vi "PCO_RecorderCopyImageCompressed.vi"(0 "phRec":u64, 1 "phCam":u64, 2 "dwImgIdx":u32, 3 "wRoiX0":u16, 4 "wRoiY0":u16, 5 "wRoiX1":u16, 6 "wRoiY1":u16, 7 "error in (no error)":errorcluster {"code" format="%x"}) -> (16 "strTimestamp":T2 {"lvTimestamp" format="%<%.6X\n%x>T"}, 17 "strMetadata":T1, 20 "phRec out":u64, 21 "ErrorMessage":i32 format="%x", 22 "bImgBuf":u8[][](array[numeric]), 23 "dwImgNumber":u32, 27 "error out":errorcluster {"code" format="%x"})   [LabVIEW 2020, in "Recorder.lvlib"]
doc: "int WINAPI PCO_RecorderCopyImageCompressed(HANDLE phRec, HANDLE phCam, DWORD dwImgIdx, WORD wRoiX0, WORD wRoiY0, WORD wRoiX1, WORD wRoiY1, BYTE* bImgBuf, DWORD* dwImgNumber,\n PCO_METADATA_STRUCT* strMetadata, PCO_TIMESTAMP_STRUCT* strTimestamp);"
uses:
  Recorder.lvlib
  LVDateTimeRec.ctl
  Structures.lvlib
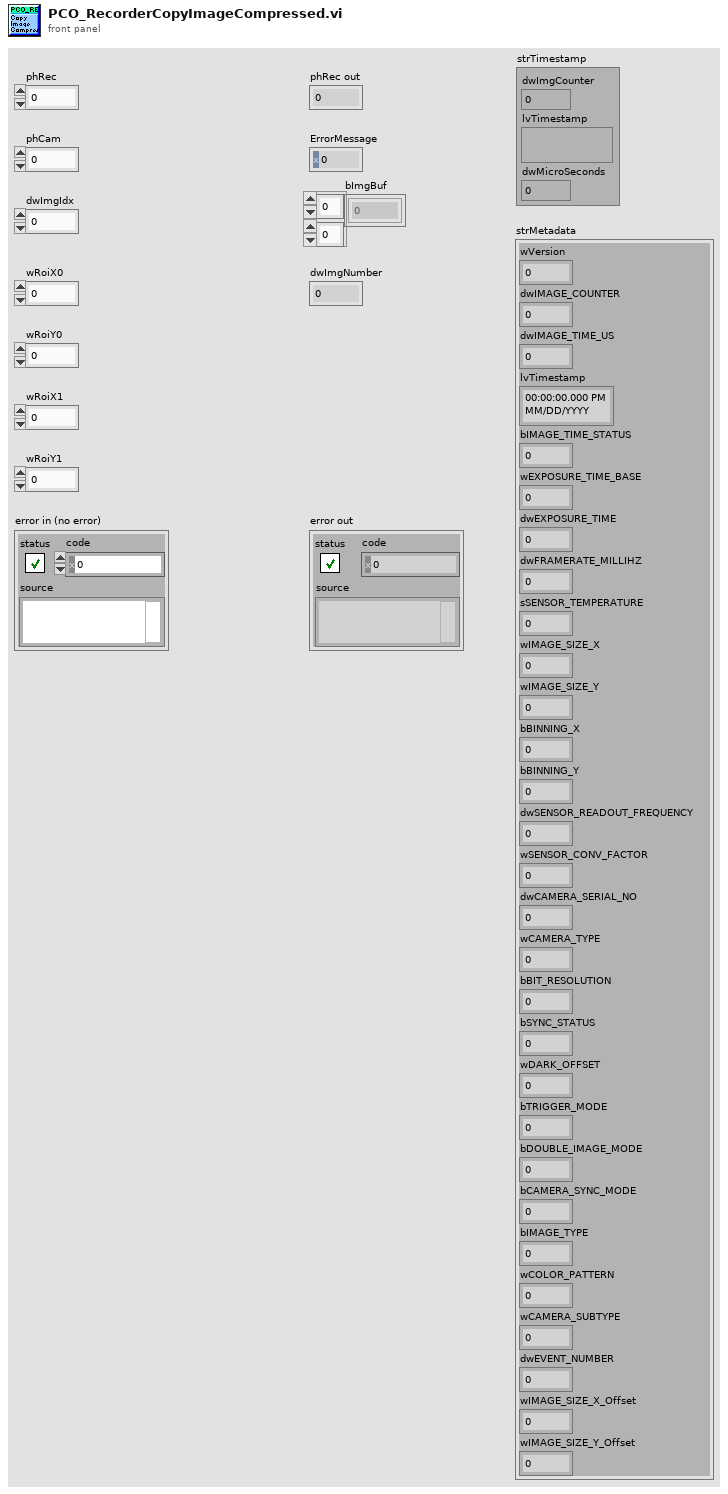
[diagram p1: front panel]
types:
  T1 = cluster{"wVersion":u16, "dwIMAGE_COUNTER":u32, "dwIMAGE_TIME_US":u32, "lvTimestamp":timestamp, "bIMAGE_TIME_STATUS":u8, "wEXPOSURE_TIME_BASE":u16, "dwEXPOSURE_TIME":u32, "dwFRAMERATE_MILLIHZ":u32, "sSENSOR_TEMPERATURE":i16, "wIMAGE_SIZE_X":u16, "wIMAGE_SIZE_Y":u16, "bBINNING_X":u8, "bBINNING_Y":u8, "dwSENSOR_READOUT_FREQUENCY":u32, "wSENSOR_CONV_FACTOR":u16, "dwCAMERA_SERIAL_NO":u32, "wCAMERA_TYPE":u16, "bBIT_RESOLUTION":u8, "bSYNC_STATUS":u8, "wDARK_OFFSET":u16, "bTRIGGER_MODE":u8, "bDOUBLE_IMAGE_MODE":u8, "bCAMERA_SYNC_MODE":u8, "bIMAGE_TYPE":u8, "wCOLOR_PATTERN":u16, "wCAMERA_SUBTYPE":u16, "dwEVENT_NUMBER":u32, "wIMAGE_SIZE_X_Offset":u16, "wIMAGE_SIZE_Y_Offset":u16}
  T2 = cluster{"dwImgCounter":u32, "lvTimestamp":timestamp, "dwMicroSeconds":u32}
  T3 = enum16{"big-endian, network order", "native, host order", "little-endian"}
  T4 = typedef "LVDateTimeRec.ctl" = cluster{"fractional second":dbl, "second":i32, "minute":i32, "hour":i32, "day of month":i32, "month":i32, "year":i32, "day of week":i32, "day of year":i32, "DST":i32}
  T5 = cluster{"wSize":u16, "dwImgCounter":u32, "wYear":u16, "wMonth":u16, "wDay":u16, "wHour":u16, "wMinute":u16, "wSecond":u16, "dwMicroSeconds":u32}
  T6 = cluster{"wSize":u16, "wVersion":u16, "bIMAGE_COUNTER_BCD":cluster{u8, u8, u8, u8}, "bIMAGE_TIME_US_BCD":cluster{u8, u8, u8}, "bIMAGE_TIME_SEC_BCD":u8, "bIMAGE_TIME_MIN_BCD":u8, "bIMAGE_TIME_HOUR_BCD":u8, "bIMAGE_TIME_DAY_BCD":u8, "bIMAGE_TIME_MON_BCD":u8, "bIMAGE_TIME_YEAR_BCD":u8, "bIMAGE_TIME_STATUS":u8, "wEXPOSURE_TIME_BASE":u16, "dwEXPOSURE_TIME":u32, "dwFRAMERATE_MILLIHZ":u32, "sSENSOR_TEMPERATURE":i16, "wIMAGE_SIZE_X":u16, "wIMAGE_SIZE_Y":u16, "bBINNING_X":u8, "bBINNING_Y":u8, "dwSENSOR_READOUT_FREQUENCY":u32, "wSENSOR_CONV_FACTOR":u16, "dwCAMERA_SERIAL_NO":u32, "wCAMERA_TYPE":u16, "bBIT_RESOLUTION":u8, "bSYNC_STATUS":u8, "wDARK_OFFSET":u16, "bTRIGGER_MODE":u8, "bDOUBLE_IMAGE_MODE":u8, "bCAMERA_SYNC_MODE":u8, "bIMAGE_TYPE":u8, "wCOLOR_PATTERN":u16, "wCAMERA_SUBTYPE":u16, "dwEVENT_NUMBER":u32, "wIMAGE_SIZE_X_Offset":u16, "wIMAGE_SIZE_Y_Offset":u16}
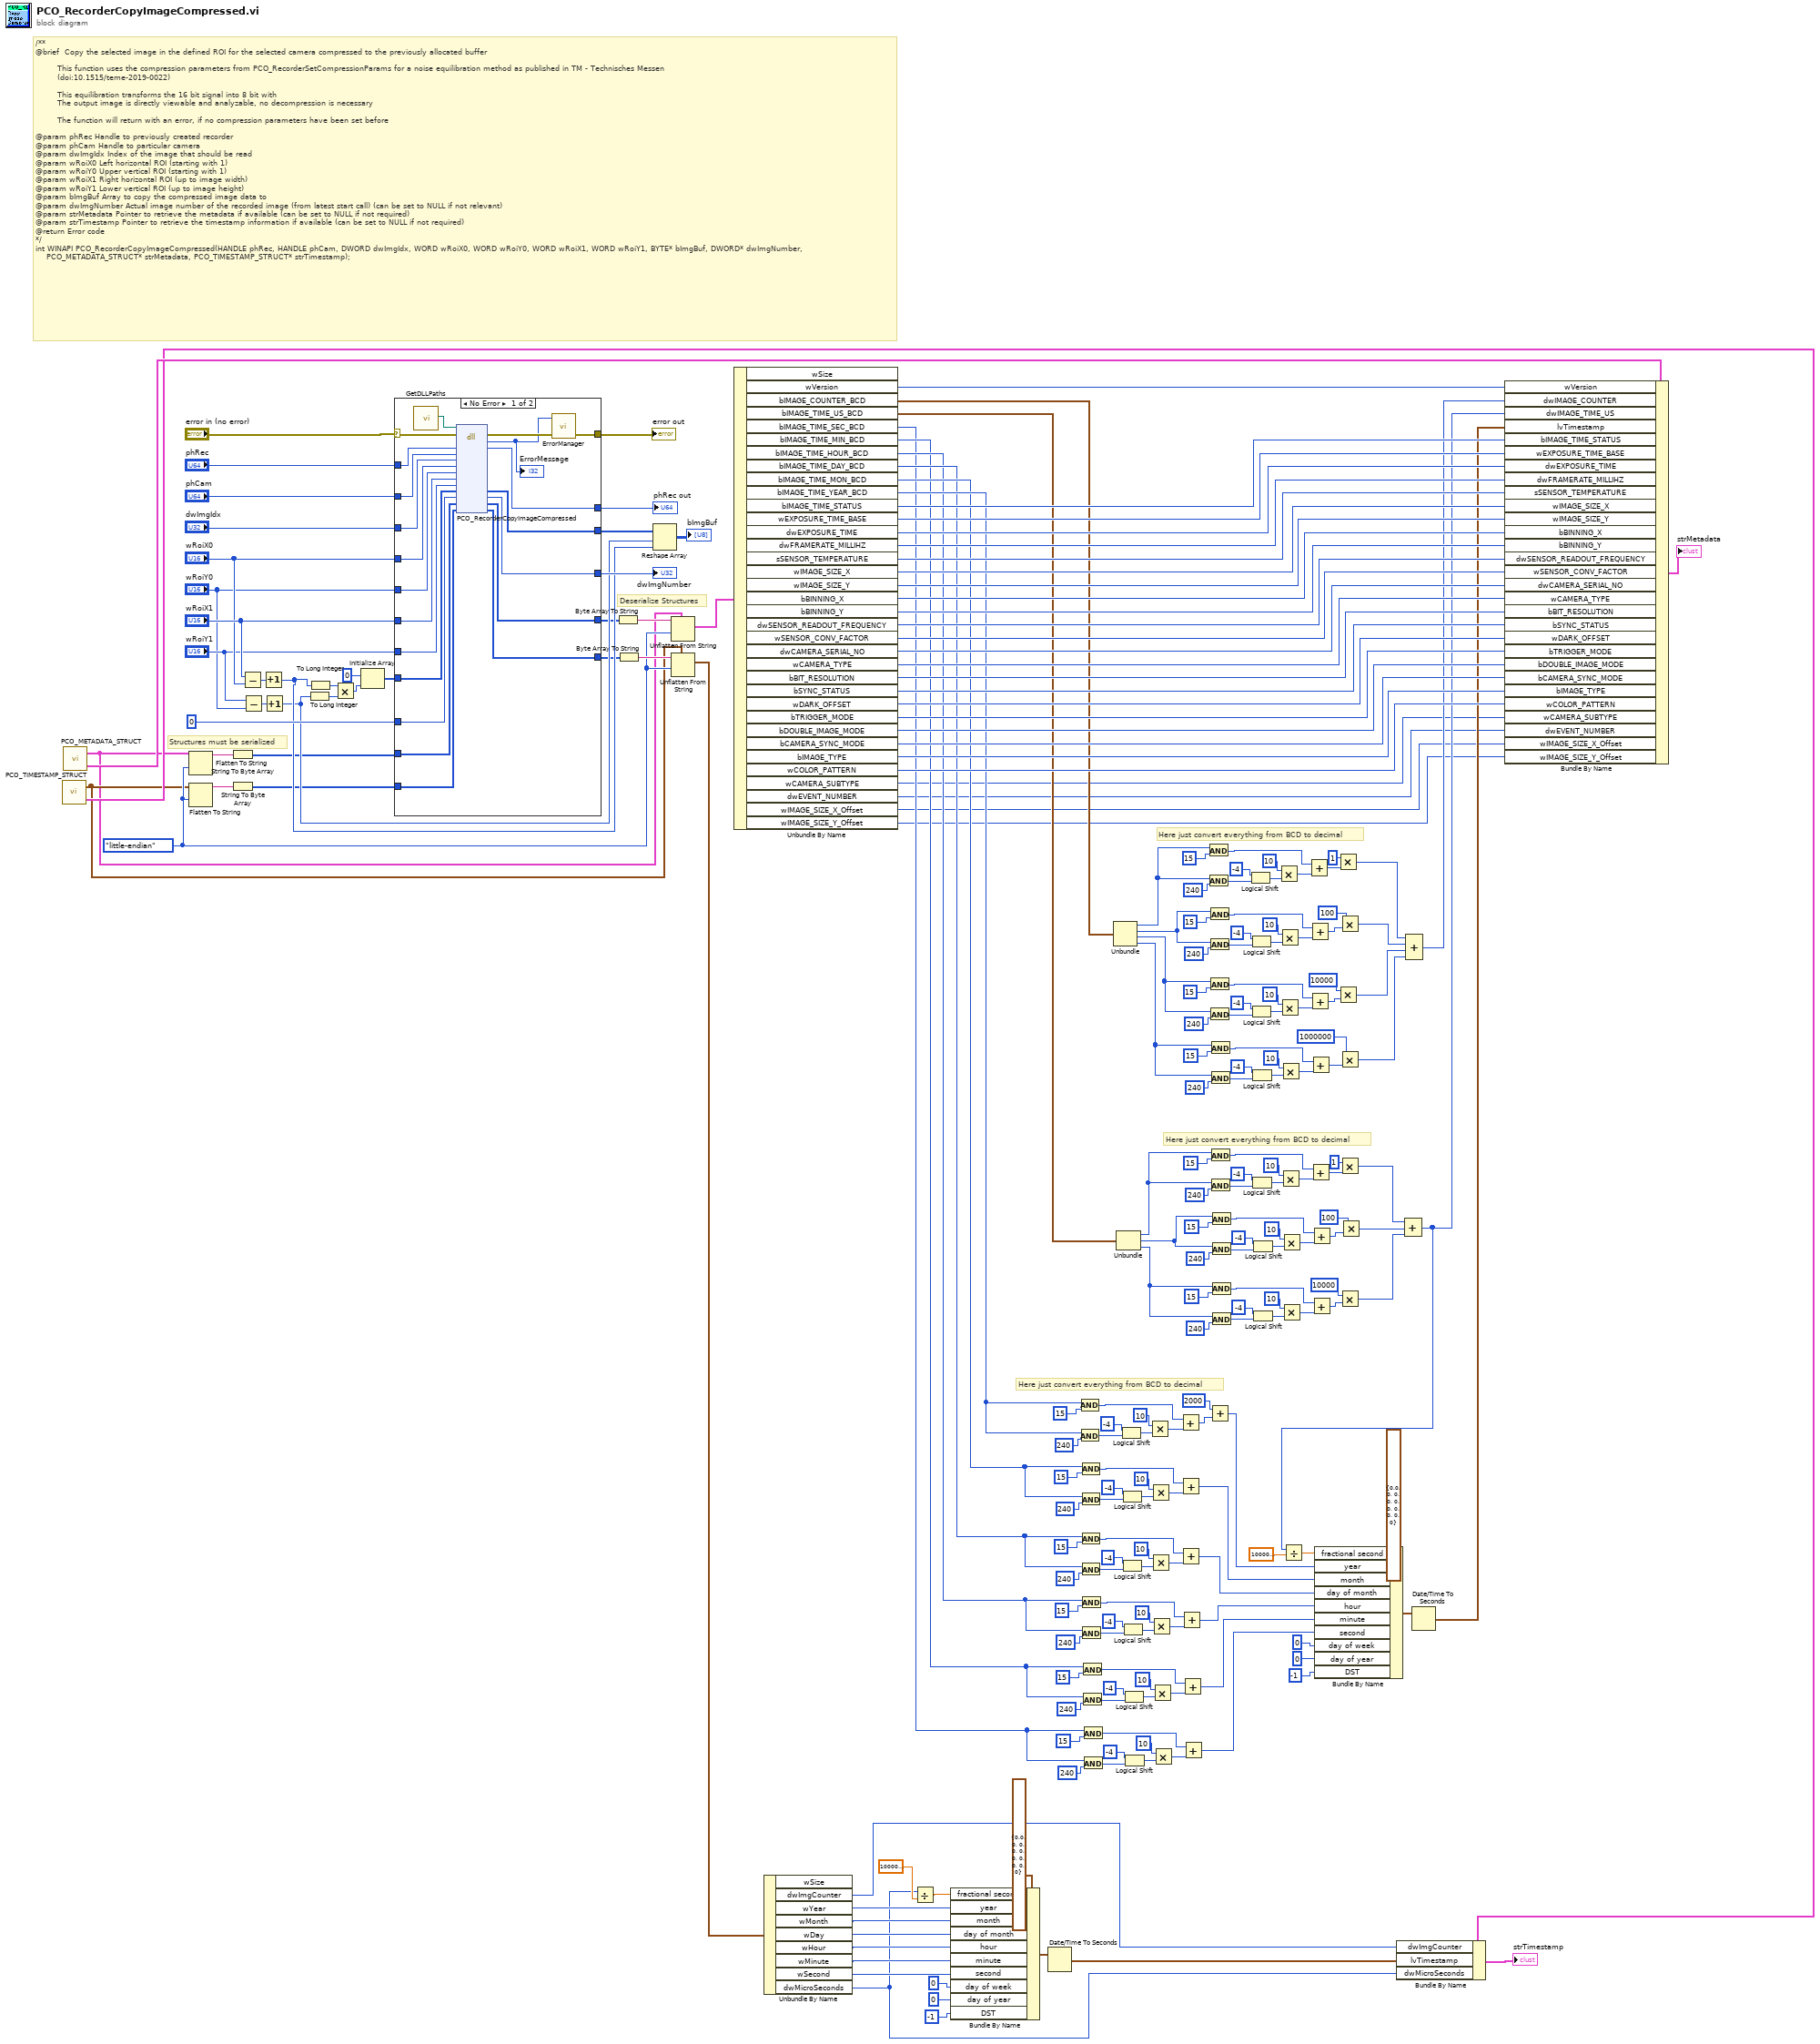
[diagram p0: block diagram]
diagram:
  w17 = T3."little-endian" ("Byte-Reihenfolge (0:Big-Endian, Netzwerkreihenfolge)")
  # "Deserialize Structures"
  # "Structures must be serialized"
  # "Here just convert everything from BCD to decimal"
  # "Here just convert everything from BCD to decimal"
  # "Here just convert everything from BCD to decimal"
  # "/**\n@brief  Copy the selected image in the defined ROI for the selected camera compressed to the previously allocated buffer\n\n        This function uses the compression parameters from PCO_RecorderSetCompressionParams for a noise equilibration method as published in TM - Technisches Messen \n        (doi:10.1515/teme-2019-0022)\n\n        This equilibration transforms the 16 bit signal into 8 bit with \n        The output image is directly viewable and analyzable, no decompression is necessary\n\n        The function will return with an error, if no compression parameters have been set before\n\n@param phRec Handle to previously created recorder\n@param phCam Handle to particular camera\n@param dwImgIdx Index of the image that should be read\n@param wRoiX0 Left horizontal ROI (starting with 1)\n@param wRoiY0 Upper vertical ROI (starting with 1)\n@param wRoiX1 Right horizontal ROI (up to image width)\n@param wRoiY1 Lower vertical ROI (up to image height)\n@param bImgBuf Array to copy the compressed image data to\n@param dwImgNumber Actual image number of the recorded image (from latest start call) (can be set to NULL if not relevant)\n@param strMetadata Pointer to retrieve the metadata if available (can be set to NULL if not required)\n@param strTimestamp Pointer to retrieve the timestamp information if available (can be set to NULL if not required)\n@return Error code\n*/\nint WINAPI PCO_RecorderCopyImageCompressed(HANDLE phRec, HANDLE phCam, DWORD dwImgIdx, WORD wRoiX0, WORD wRoiY0, WORD wRoiX1, WORD wRoiY1, BYTE* bImgBuf, DWORD* dwImgNumber,\n    PCO_METADATA_STRUCT* strMetadata, PCO_TIMESTAMP_STRUCT* strTimestamp);"
  n1 = call "PCO_TIMESTAMP_STRUCT.vi"() -> ("PCO_TIMESTAMP_STRUCT"=w218:T2, "PCO_TIMESTAMP_STRUCT_Raw"=w16:T5)  [unwired: 4 in, 2 out]
  n2 = call "PCO_METADATA_STRUCT.vi"() -> ("PCO_METADATA_STRUCT"=w223:T1, "PCO_METADATA_STRUCT_Raw"=w15:T6)  [unwired: 4 in, 2 out]
  n3 = Flatten To String(anything=w15, byte order (0:big-endian, network order)=w17) -> (data string=w25:string)  [unwired: 2 in, 2 out]
  n4 = Flatten To String(anything=w16, byte order (0:big-endian, network order)=w17) -> (data string=w27:string)  [unwired: 2 in, 2 out]
  n5 = String To Byte Array(string=w25) -> (unsigned byte array=w24:u8[])
  n6 = String To Byte Array(string=w27) -> (unsigned byte array=w26:u8[])
  n7 = Subtract(x="wRoiX1", y="wRoiX0") -> (x-y=w228:u16)
  n8 = Subtract(x="wRoiY1", y="wRoiY0") -> (x-y=w225:u16)
  n9 = Increment(x=w228) -> (x+1=w29:u16)
  n10 = Increment(x=w225) -> (x+1=w28:u16)
  n11 = To Long Integer(number=w28) -> (32bit integer=w31:i32)
  n12 = To Long Integer(number=w29) -> (32bit integer=w30:i32)
  n13 = Multiply(x=w30, y=w31) -> (x*y=w224:i32)
  n14 = Initialize Array(u8 0 ("element"), w224) -> (w236:u8[])
  n15 = case shown="No Error" "error in (no error)" {
    selector: "error in (no error)" -> [w248 w267]
    tunnel: "phRec" -> [w261 w266]
    tunnel: [w260 w266] -> w239
    tunnel: "phCam" -> [w259 _]
    tunnel: "dwImgIdx" -> [w258 _]
    tunnel: "wRoiX0" -> [w257 _]
    tunnel: "wRoiY0" -> [w256 _]
    tunnel: "wRoiX1" -> [w255 _]
    tunnel: "wRoiY1" -> [w254 _]
    tunnel: w236 -> [w253 w265]
    tunnel: [w252 w265] -> w33
    tunnel: [w251 w264] -> w234
    tunnel: [w250 w263] -> w23
    tunnel: [w249 w262] -> w22
    tunnel: [w247 w267] -> w233
    tunnel: w26 -> [w244 w262]
    tunnel: w24 -> [w243 w263]
    tunnel: u32 0 ("dwImgNumber") -> [w242 w264]
    frame No Error {
      n16 = call "GetDLLPaths.vi"() -> ("PCO_Recorder_Path"=w241:path)  [unwired: 9 in, 2 out]
      n17 = dll-call lib="?" fn="PCO_RecorderCopyImageCompressed"(path in=w241, error in=w248, "phRec"=w261, "phCam"=w259, "dwImgIdx"=w258, "wRoiX0"=w257, "wRoiY0"=w256, "wRoiX1"=w255, "wRoiY1"=w254, "bImgBuf"=w253, "dwImgNumber"=w242, "strMetadata"=w243, "strTimestamp"=w244) -> (error out=w246:errorcluster, "return type"=w245:i32, "phRec"=w260:u64, "bImgBuf"=w252:u8[], "dwImgNumber"=w251:u32, "strMetadata"=w250:u8[], "strTimestamp"=w249:u8[])  [unwired: 7 in, 1 out]
      "ErrorMessage" <- w245
      n18 = call "ErrorManager.vi"("error in (no error)"=w246, "error code"=w245) -> ("error out"=w247:errorcluster)  [unwired: 3 in]
    }
    frame Error {
    }
  }
  "phRec out" <- w239
  "dwImgNumber" <- w234
  "error out" <- w233
  n19 = Byte Array To String(unsigned byte array=w23) -> (string=w21:string)
  n20 = Byte Array To String(unsigned byte array=w22) -> (string=w20:string)
  n21 = Reshape Array(w33, w28, w29) -> (→"bImgBuf":u8[][])
  n22 = Unflatten From String(type=w15, binary string=w21, byte order (0:big-endian, network order)=w17) -> (value=w19:T6)  [unwired: 2 in, 2 out]
  n23 = Unflatten From String(type=w16, binary string=w20, byte order (0:big-endian, network order)=w17) -> (value=w18:T5)  [unwired: 2 in, 2 out]
  n24 = Unbundle By Name(w19) -> ("wVersion"=w222:u16, "bIMAGE_COUNTER_BCD"=w120:cluster{u8, u8, u8, u8}, "bIMAGE_TIME_US_BCD"=w42:cluster{u8, u8, u8}, "bIMAGE_TIME_SEC_BCD"=w132:u8, "bIMAGE_TIME_MIN_BCD"=w133:u8, "bIMAGE_TIME_HOUR_BCD"=w134:u8, "bIMAGE_TIME_DAY_BCD"=w135:u8, "bIMAGE_TIME_MON_BCD"=w136:u8, "bIMAGE_TIME_YEAR_BCD"=w181:u8, "bIMAGE_TIME_STATUS"=w203:u8, "wEXPOSURE_TIME_BASE"=w202:u16, "dwEXPOSURE_TIME"=w201:u32, "dwFRAMERATE_MILLIHZ"=w200:u32, "sSENSOR_TEMPERATURE"=w199:i16, "wIMAGE_SIZE_X"=w198:u16, "wIMAGE_SIZE_Y"=w197:u16, "bBINNING_X"=w196:u8, "bBINNING_Y"=w195:u8, "dwSENSOR_READOUT_FREQUENCY"=w194:u32, "wSENSOR_CONV_FACTOR"=w193:u16, "dwCAMERA_SERIAL_NO"=w192:u32, "wCAMERA_TYPE"=w191:u16, "bBIT_RESOLUTION"=w190:u8, "bSYNC_STATUS"=w189:u8, "wDARK_OFFSET"=w188:u16, "bTRIGGER_MODE"=w187:u8, "bDOUBLE_IMAGE_MODE"=w186:u8, "bCAMERA_SYNC_MODE"=w185:u8, "bIMAGE_TYPE"=w184:u8, "wCOLOR_PATTERN"=w183:u16, "wCAMERA_SUBTYPE"=w4:u16, "dwEVENT_NUMBER"=w3:u32, "wIMAGE_SIZE_X_Offset"=w2:u16, "wIMAGE_SIZE_Y_Offset"=w1:u16)  [unwired: 1 out]
  n25 = Unbundle By Name(w18) -> ("dwImgCounter"=w205:u32, "wYear"=w207:u16, "wMonth"=w208:u16, "wDay"=w209:u16, "wHour"=w210:u16, "wMinute"=w211:u16, "wSecond"=w212:u16, "dwMicroSeconds"=w13:u32)  [unwired: 1 out]
  n26 = Divide(x=w13, y=1000000.0 ("fractional second")) -> (x/y=w12:dbl)
  n27 = Bundle By Name(cluster=T4 {"fractional second"=0.0, "second"=0, "minute"=0, "hour"=0, "day of month"=0, "month"=0, "year"=0, "day of week"=0, "day of year"=0, "DST"=0} ("date time rec"), "fractional second"=w12, "year"=w207, "month"=w208, "day of month"=w209, "hour"=w210, "minute"=w211, "second"=w212, "day of week"=0, "day of year"=0, "DST"=-1) -> (w217:T4)
  n28 = Date/Time To Seconds(2:w217) -> (0:w206:timestamp)  [unwired: 1 in]
  n29 = And(x=w181, y=u8 15) -> (x .and. y?=w177:u8)
  n30 = And(x=w181, y=u8 240) -> (x .and. y?=w219:u8)
  n31 = And(x=w136, y=u8 15) -> (x .and. y?=w176:u8)
  n32 = And(x=w136, y=u8 240) -> (x .and. y?=w171:u8)
  n33 = And(x=w135, y=u8 15) -> (x .and. y?=w160:u8)
  n34 = And(x=w135, y=u8 240) -> (x .and. y?=w155:u8)
  n35 = And(x=w134, y=u8 15) -> (x .and. y?=w161:u8)
  n36 = And(x=w134, y=u8 240) -> (x .and. y?=w166:u8)
  n37 = And(x=w133, y=u8 15) -> (x .and. y?=w145:u8)
  n38 = And(x=w133, y=u8 240) -> (x .and. y?=w150:u8)
  n39 = And(x=w132, y=u8 15) -> (x .and. y?=w144:u8)
  n40 = And(x=w132, y=u8 240) -> (x .and. y?=w139:u8)
  n41 = Unbundle(w120) -> (w50:u8, w49:u8, w48:u8, w47:u8)
  n42 = Unbundle(w42) -> (w41:u8, w40:u8, w39:u8)
  n43 = Logical Shift(y=i16 -4, x=w219) -> (x << y=w180:u8)
  n44 = Logical Shift(y=i16 -4, x=w171) -> (x << y=w173:u8)
  n45 = Logical Shift(y=i16 -4, x=w155) -> (x << y=w157:u8)
  n46 = Logical Shift(y=i16 -4, x=w166) -> (x << y=w164:u8)
  n47 = Logical Shift(y=i16 -4, x=w150) -> (x << y=w148:u8)
  n48 = Logical Shift(y=i16 -4, x=w139) -> (x << y=w141:u8)
  n49 = Multiply(x=u8 10, y=w180) -> (x*y=w178:u8)
  n50 = Multiply(x=u8 10, y=w173) -> (x*y=w175:u8)
  n51 = Multiply(x=u8 10, y=w157) -> (x*y=w159:u8)
  n52 = Multiply(x=u8 10, y=w164) -> (x*y=w162:u8)
  n53 = Multiply(x=u8 10, y=w148) -> (x*y=w146:u8)
  n54 = Multiply(x=u8 10, y=w141) -> (x*y=w143:u8)
  n55 = Add(x=w177, y=w178) -> (x+y=w11:u8)
  n56 = Add(x=w176, y=w175) -> (x+y=w126:u8)
  n57 = Add(x=w160, y=w159) -> (x+y=w125:u8)
  n58 = Add(x=w161, y=w162) -> (x+y=w124:u8)
  n59 = Add(x=w145, y=w146) -> (x+y=w123:u8)
  n60 = Add(x=w144, y=w143) -> (x+y=w122:u8)
  n61 = And(x=w50, y=u8 15) -> (x .and. y?=w95:u8)
  n62 = And(x=w50, y=u8 240) -> (x .and. y?=w90:u8)
  n63 = And(x=w49, y=u8 15) -> (x .and. y?=w96:u8)
  n64 = And(x=w49, y=u8 240) -> (x .and. y?=w101:u8)
  n65 = And(x=w48, y=u8 15) -> (x .and. y?=w112:u8)
  n66 = And(x=w48, y=u8 240) -> (x .and. y?=w117:u8)
  n67 = Add(x=2000, y=w11) -> (x+y=w9:i32)
  n68 = And(x=w47, y=u8 15) -> (x .and. y?=w111:u8)
  n69 = And(x=w47, y=u8 240) -> (x .and. y?=w106:u8)
  n70 = And(x=w41, y=u8 15) -> (x .and. y?=w66:u8)
  n71 = And(x=w41, y=u8 240) -> (x .and. y?=w71:u8)
  n72 = And(x=w40, y=u8 15) -> (x .and. y?=w65:u8)
  n73 = And(x=w40, y=u8 240) -> (x .and. y?=w60:u8)
  n74 = And(x=w39, y=u8 15) -> (x .and. y?=w57:u8)
  n75 = And(x=w39, y=u8 240) -> (x .and. y?=w52:u8)
  n76 = Logical Shift(y=i16 -4, x=w90) -> (x << y=w92:u8)
  n77 = Logical Shift(y=i16 -4, x=w101) -> (x << y=w99:u8)
  n78 = Logical Shift(y=i16 -4, x=w117) -> (x << y=w115:u8)
  n79 = Logical Shift(y=i16 -4, x=w106) -> (x << y=w108:u8)
  n80 = Logical Shift(y=i16 -4, x=w71) -> (x << y=w69:u8)
  n81 = Logical Shift(y=i16 -4, x=w60) -> (x << y=w62:u8)
  n82 = Logical Shift(y=i16 -4, x=w52) -> (x << y=w54:u8)
  n83 = Multiply(x=u8 10, y=w92) -> (x*y=w94:u8)
  n84 = Multiply(x=u8 10, y=w99) -> (x*y=w97:u8)
  n85 = Multiply(x=u8 10, y=w115) -> (x*y=w113:u8)
  n86 = Multiply(x=u8 10, y=w108) -> (x*y=w110:u8)
  n87 = Multiply(x=u8 10, y=w69) -> (x*y=w67:u8)
  n88 = Multiply(x=u8 10, y=w62) -> (x*y=w64:u8)
  n89 = Multiply(x=u8 10, y=w54) -> (x*y=w56:u8)
  n90 = Add(x=w95, y=w94) -> (x+y=w84:u8)
  n91 = Add(x=w96, y=w97) -> (x+y=w87:u8)
  n92 = Add(x=w112, y=w113) -> (x+y=w86:u8)
  n93 = Add(x=w111, y=w110) -> (x+y=w85:u8)
  n94 = Add(x=w66, y=w67) -> (x+y=w76:u8)
  n95 = Add(x=w65, y=w64) -> (x+y=w74:u8)
  n96 = Add(x=w57, y=w56) -> (x+y=w75:u8)
  n97 = Multiply(x=u32 1, y=w84) -> (x*y=w46:u32)
  n98 = Multiply(x=u32 10000, y=w86) -> (x*y=w44:u32)
  n99 = Multiply(x=u32 100, y=w87) -> (x*y=w45:u32)
  n100 = Multiply(x=u32 1000000, y=w85) -> (x*y=w43:u32)
  n101 = Multiply(x=u32 1, y=w76) -> (x*y=w37:u32)
  n102 = Multiply(x=u32 10000, y=w75) -> (x*y=w35:u32)
  n103 = Multiply(x=u32 100, y=w74) -> (x*y=w36:u32)
  n104 = Bundle By Name(cluster=w218, "dwImgCounter"=w205, "lvTimestamp"=w206, "dwMicroSeconds"=w13) -> (→"strTimestamp":T2)
  n105 = Compound Arithmetic op=ADD(w37, w36, w35) -> (w7:u32)
  n106 = Divide(x=w7, y=1000000.0 ("fractional second")) -> (x/y=w6:dbl)
  n107 = Bundle By Name(cluster=T4 {"fractional second"=0.0, "second"=0, "minute"=0, "hour"=0, "day of month"=0, "month"=0, "year"=0, "day of week"=0, "day of year"=0, "DST"=0} ("date time rec"), "fractional second"=w6, "year"=w9, "month"=w126, "day of month"=w125, "hour"=w124, "minute"=w123, "second"=w122, "day of week"=0, "day of year"=0, "DST"=-1) -> (w127:T4)
  n108 = Compound Arithmetic op=ADD(w46, w45, w44, w43) -> (w34:u32)
  n109 = Date/Time To Seconds(2:w127) -> (0:w121:timestamp)  [unwired: 1 in]
  n110 = Bundle By Name(cluster=w223, "wVersion"=w222, "dwIMAGE_COUNTER"=w34, "dwIMAGE_TIME_US"=w7, "lvTimestamp"=w121, "bIMAGE_TIME_STATUS"=w203, "wEXPOSURE_TIME_BASE"=w202, "dwEXPOSURE_TIME"=w201, "dwFRAMERATE_MILLIHZ"=w200, "sSENSOR_TEMPERATURE"=w199, "wIMAGE_SIZE_X"=w198, "wIMAGE_SIZE_Y"=w197, "bBINNING_X"=w196, "bBINNING_Y"=w195, "dwSENSOR_READOUT_FREQUENCY"=w194, "wSENSOR_CONV_FACTOR"=w193, "dwCAMERA_SERIAL_NO"=w192, "wCAMERA_TYPE"=w191, "bBIT_RESOLUTION"=w190, "bSYNC_STATUS"=w189, "wDARK_OFFSET"=w188, "bTRIGGER_MODE"=w187, "bDOUBLE_IMAGE_MODE"=w186, "bCAMERA_SYNC_MODE"=w185, "bIMAGE_TYPE"=w184, "wCOLOR_PATTERN"=w183, "wCAMERA_SUBTYPE"=w4, "dwEVENT_NUMBER"=w3, "wIMAGE_SIZE_X_Offset"=w2, "wIMAGE_SIZE_Y_Offset"=w1) -> (→"strMetadata":T1)
